vi "slopes_processors_list.vi"() -> ()   [LabVIEW 2020]
uses:
  SlopesPostProcessorList.lvclass
  HasoSlopes.lvclass
  HasoData.lvclass
panel:
  in  "Output Haso slopes files base name":string="Data\\data_phase_computation_processed_"
  out "Processed slopes computed and saved":bool
  out "Reference slopes loaded":bool
  out "Input slopes loaded":bool
  in  "Input Reference slopes file name":string="Data\\data_phase_computation.has"
  in  "Input Haso slopes files base name":string="Data\\data_phase_computation_"
  out "error out":errorcluster
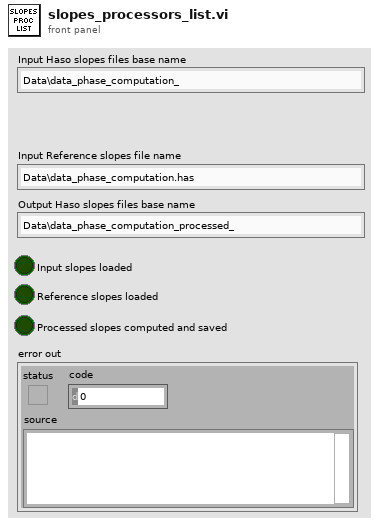
[diagram p1: front panel]
types:
  T1 = typedef "DataHaso acquisition information.ctl" = cluster{"HASO information":T2, "Acquisition information":T3, "SLOPES ENGINE information":T8, "Source wavelength (nm)":dbl, "FillPercent_%":dbl, "session_name":string}
  T2 = typedef "HASO information.ctl" = cluster{"HASO serial number":string, "HASO model":string, "Lower calibration wavelength (nm)":dbl, "Upper calibration wavelength (nm)":dbl, "Revision":i32}
  T3 = typedef "Image information.ctl" = cluster{"Image general information":T4, "Acquisition information":T5, "Number of pixels":T6, "Number of bits":T7}
  T4 = typedef "Image general information.ctl" = cluster{"Camera serial number":string, "Smearing removed":bool, "Background image removed":bool, "Time Stamp":timestamp, "Comment":string, "Camera_MAX_Level":i32}
  T5 = typedef "Image acquisition information.ctl" = cluster{"Exposure duration (us)":i32, "Exposure duration specified (us)":i32, "Gain":sgl, "Number of summed images":i32, "Trigger type":string}
  T6 = typedef "Point2D.ctl" = cluster{"X":u32, "Y":u32}
  T7 = typedef "Data alignment enum.ctl" = enum16{"8", "16", "32"}
  T8 = typedef "SlopesEngineSetup.ctl" = cluster{"Start sub-aperture":T6, "Pupil average":dbl}
  T9 = typedef "Point2Df.ctl" = cluster{"X":sgl, "Y":sgl}
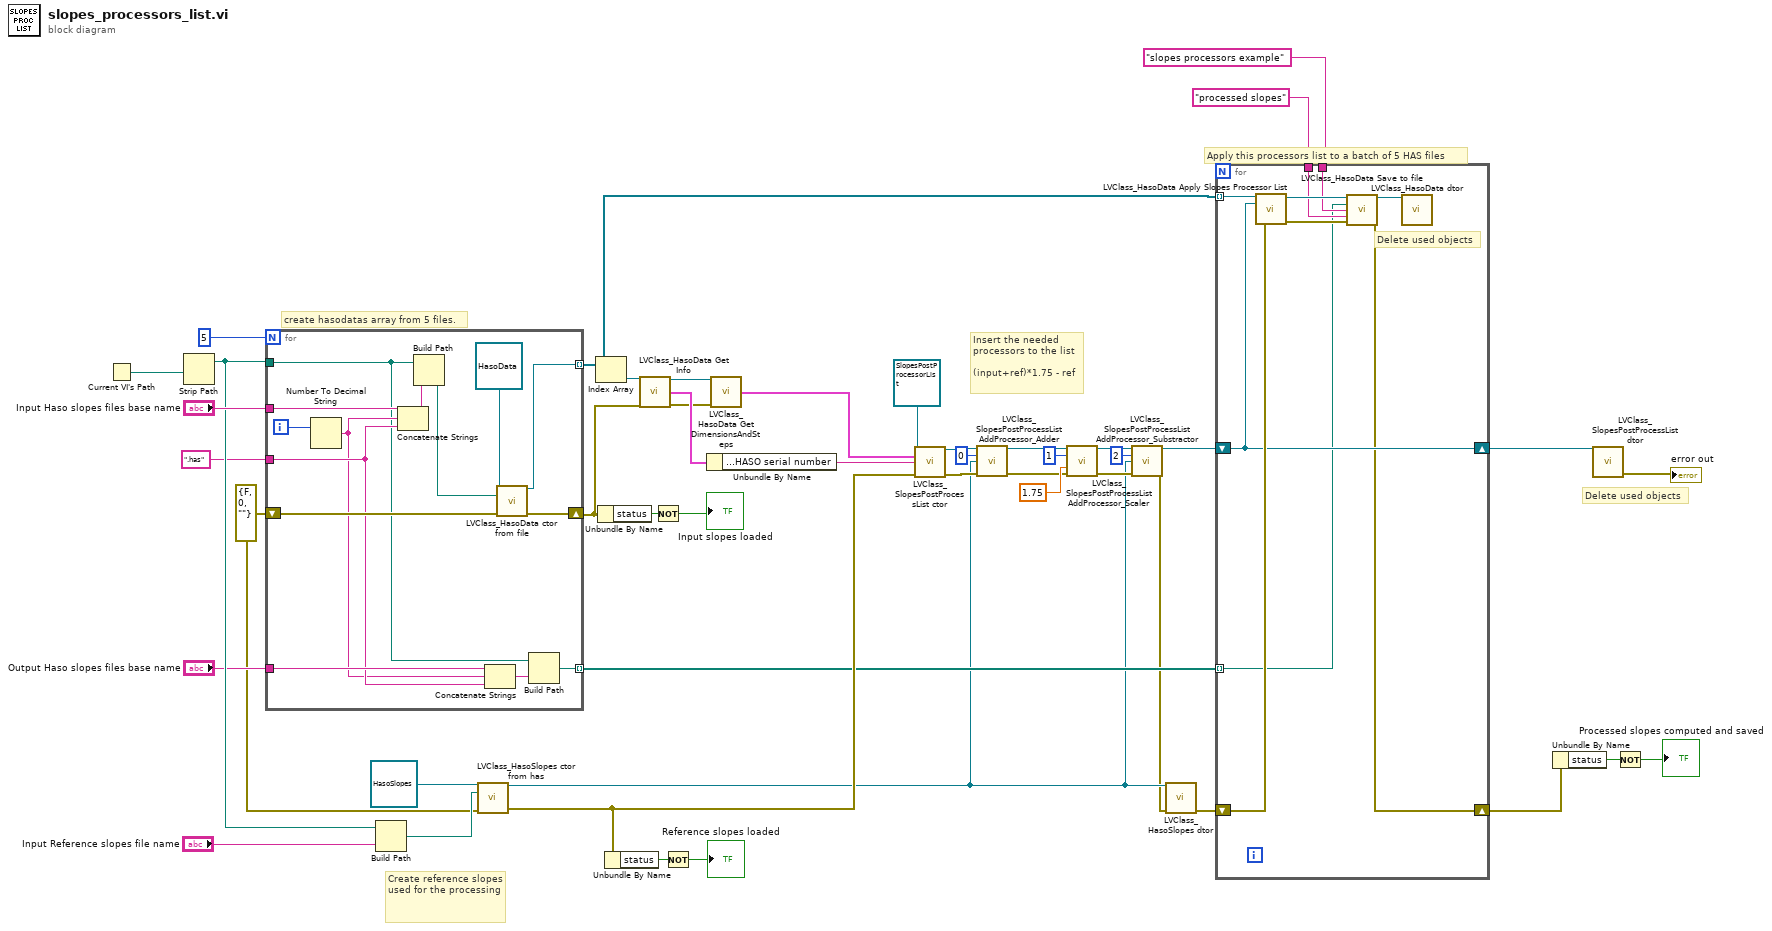
[diagram p0: block diagram]
diagram:
  w6 = errorcluster {"status"=FALSE, "code"=0, "source"=""} ("error out")
  # "Delete used objects"
  # "Apply this processors list to a batch of 5 HAS files"
  # "Insert the needed\nprocessors to the list\n\n(input+ref)*1.75 - ref"
  # "Create reference slopes used for the processing"
  # "create hasodatas array from 5 files."
  n1 = Current VI's Path() -> (path=w28:path)
  n2 = Strip Path(path=w28) -> (stripped path=w9:path)  [unwired: 1 out]
  n3 = for {
    N: 5 -> [_]
    tunnel: w9 -> [w49]
    tunnel: [w57] -> w12 mode=indexing
    shift-right: [w55] -> w24
    shift-left: w6 -> [w54]
    tunnel: ".has" ("Haso slopes files extension") -> [w51]
    tunnel: "Input Haso slopes files base name" -> [w53]
    tunnel: "Output Haso slopes files base name" -> [w52]
    tunnel: [w47] -> w7 mode=indexing
    i -> [w60]
    n4 = Number To Decimal String(number=w60) -> (decimal integer string=w50:string)  [unwired: 1 in]
    n5 = Concatenate Strings(w53, w50, w51) -> (w59:string)
    n6 = Build Path(base path=w49, name or relative path=w59) -> (appended path=w58:path)
    n7 = Concatenate Strings(w52, w50, w51) -> (w48:string)
    n8 = call "LVClass_HasoData ctor from file.vi"("HasoData in"=refnum<class "HasoData.lvclass"> refnum, "HAS file path"=w58, "error in (no error)"=w54) -> ("HasoData out"=w57:refnum<class "HasoData.lvclass">, "error out"=w55:errorcluster)  [unwired: 11 in]
    n9 = Build Path(base path=w49, name or relative path=w48) -> (appended path=w47:path)
  }
  n10 = Build Path(base path=w9, name or relative path="Input Reference slopes file name") -> (appended path=w26:path)
  n11 = call "LVClass_HasoSlopes ctor from has.vi"("HasoSlopes in"=refnum<class "HasoSlopes.lvclass"> refnum, ".has path"=w26, "error in (no error)"=w6) -> ("HasoSlopes out"=w3:refnum<class "HasoSlopes.lvclass">, "error out"=w22:errorcluster)  [unwired: 11 in]
  n12 = Index Array(array=w12) -> (element=w45:refnum<class "HasoData.lvclass">)  [unwired: 1 in]
  n13 = Unbundle By Name(w24) -> ("status"=w14:bool)
  n14 = Unbundle By Name(w22) -> ("status"=w18:bool)
  n15 = call "LVClass_HasoData Get Info.vi"("HasoData in"=w45, "error in (no error)"=w24) -> ("HasoData out"=w25:refnum<class "HasoData.lvclass">, "DataHaso acquisition information 2"=w46:T1, "error out"=w29:errorcluster)  [unwired: 11 in]
  n16 = Not(x=w14) -> (.not. x?=→"Input slopes loaded":bool)
  n17 = Not(x=w18) -> (.not. x?=→"Reference slopes loaded":bool)
  n18 = Unbundle By Name(w46) -> ("HASO information.HASO serial number"=w43:string)
  n19 = call "LVClass_HasoData Get DimensionsAndSteps.vi"("HasoData in"=w25, "error in (no error)"=w29) -> ("Dimensions"=w44:cluster{"size":T6, "steps":T9})  [unwired: 11 in, 2 out]
  n20 = call "LVClass_SlopesPostProcessList ctor.vi"("SlopesPostProcessorList in"=refnum<class "SlopesPostProcessorList.lvclass"> refnum, "Dimensions_um"=w44, "serial"=w43, "error in (no error)"=w22) -> ("SlopesPostProcessorList out"=w40:refnum<class "SlopesPostProcessorList.lvclass">, "error out"=w23:errorcluster)  [unwired: 10 in]
  n21 = call "LVClass_SlopesPostProcessList AddProcessor_Adder.vi"("SlopesPostProcessorList in"=w40, "Position"=0, "HasoSlopes.lvclass"=w3, "error in (no error)"=w23) -> ("SlopesPostProcessorList out"=w38:refnum<class "SlopesPostProcessorList.lvclass">, "error out"=w35:errorcluster)  [unwired: 10 in]
  n22 = call "LVClass_SlopesPostProcessList AddProcessor_Scaler.vi"("SlopesPostProcessorList in"=w38, "Position"=1, "scaler"=sgl 1.75, "error in (no error)"=w35) -> ("SlopesPostProcessorList out"=w34:refnum<class "SlopesPostProcessorList.lvclass">, "error out"=w32:errorcluster)  [unwired: 10 in]
  n23 = call "LVClass_SlopesPostProcessList AddProcessor_Substractor.vi"("SlopesPostProcessorList in"=w34, "Position"=2, "HasoSlopes.lvclass"=w3, "error in (no error)"=w32) -> ("SlopesPostProcessorList out"=w31:refnum<class "SlopesPostProcessorList.lvclass">, "error out"=w2:errorcluster)  [unwired: 10 in]
  n24 = call "LVClass_HasoSlopes dtor.vi"("HasoSlopes in"=w3, "error in (no error)"=w2) -> ("error out"=w1:errorcluster)  [unwired: 12 in, 1 out]
  n25 = for {
    tunnel: w12 -> [w70] mode=indexing
    shift-right: [w65] -> w11
    shift-left: w1 -> [w69]
    shift-right: [w68] -> w30
    shift-left: w31 -> [w68]
    tunnel: "processed slopes" -> [w64]
    tunnel: "slopes processors example" -> [w63]
    tunnel: w7 -> [w62] mode=indexing
    # "Delete used objects"
    n26 = call "LVClass_HasoData Apply Slopes Processor List.vi"("HasoData in"=w70, "SlopesPostProcessorList"=w68, "error in (no error)"=w69) -> ("HasoData out"=w66:refnum<class "HasoData.lvclass">, "error out"=w67:errorcluster)  [unwired: 11 in]
    n27 = call "LVClass_HasoData Save to file.vi"("HasoData in"=w66, "HAS file path"=w62, "session_name"=w63, "comments"=w64, "error in (no error)"=w67) -> ("HasoData out"=w61:refnum<class "HasoData.lvclass">, "error out"=w65:errorcluster)  [unwired: 9 in]
    n28 = call "LVClass_HasoData dtor.vi"("HasoData in"=w61) -> ()  [unwired: 13 in, 2 out]
  }
  n29 = Unbundle By Name(w11) -> ("status"=w16:bool)
  n30 = call "LVClass_SlopesPostProcessList dtor.vi"("SlopesPostProcessorList in"=w30) -> ("error out"=→"error out":errorcluster)  [unwired: 13 in, 1 out]
  n31 = Not(x=w16) -> (.not. x?=→"Processed slopes computed and saved":bool)
